vi "joystick_read.vi"(8 "error in (no error)":errorcluster, 10 "目标位置":dbl[](array[numeric]), 11 "Refnum in":refnum<k1>) -> (0 "error out":errorcluster, 3 "Array":dbl[](array[numeric]))   [LabVIEW 2017]
uses:
  <vilib>/Utility/inputDevices.llb/joystickAcquire.vi
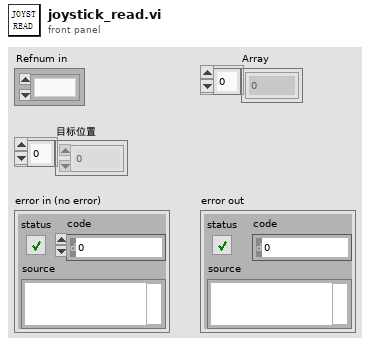
[diagram p1: front panel]
types:
  T1 = cluster{"X axis":i32, "Y axis":i32, "Z axis":i32, "X axis rotation":i32, "Y axis rotation":i32, "Z axis rotation":i32, "U axis":i32, "V axis":i32}
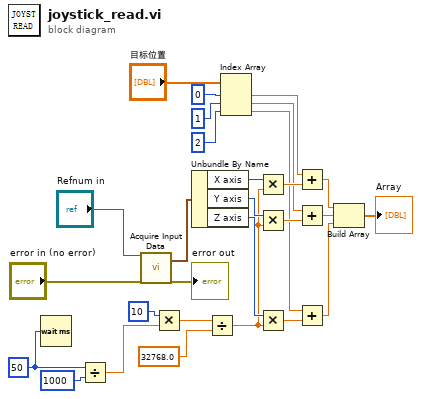
[diagram p0: block diagram]
diagram:
  w9 = 50 ("y")
  n1 = Wait (ms)(milliseconds to wait=w9) -> ()  [unwired: 1 out]
  n2 = Divide(x=w9, y=1000) -> (x/y=w12:dbl)
  n3 = call-poly <vilib>:"Acquire Input Data.vi"("device ID"="Refnum in", "error in (no error)"="error in (no error)") -> ("axis info"=w3:T1, "error out"=→"error out":errorcluster)  [unwired: 13 in, 3 out]
  n4 = Multiply(x=10 ("y"), y=w12) -> (x*y=w13:dbl)
  n5 = Unbundle By Name(w3) -> ("X axis"=w18:i32, "Y axis"=w20:i32, "Z axis"=w21:i32)
  n6 = Divide(x=w13, y=32768.0) -> (x/y=w19:dbl)
  n7 = Index Array(array="目标位置", index #1=0 ("index"), index #2=1 ("index"), index #3=2 ("index")) -> (element #1=w15:dbl, element #2=w16:dbl, element #3=w17:dbl)
  n8 = Multiply(x=w18, y=w19) -> (x*y=w22:dbl)
  n9 = Multiply(x=w20, y=w19) -> (x*y=w23:dbl)
  n10 = Multiply(x=w21, y=w19) -> (x*y=w24:dbl)
  n11 = Add(x=w15, y=w22) -> (x+y=w25:dbl)
  n12 = Add(x=w16, y=w23) -> (x+y=w26:dbl)
  n13 = Add(x=w17, y=w24) -> (x+y=w27:dbl)
  n14 = Build Array(w25, w26, w27) -> (→"Array":dbl[])
